vi "BehaviorControl.vi"() -> ()   [LabVIEW 2011]
uses:
  <instrlib>/niHWS/nihws.llb/niHWS Open File Permissions ID.ctl
  <vilib>/DAQmx/read.llb/DAQmx Read (Analog 1D Wfm NChan NSamp).vi
  <vilib>/DAQmx/create/channels.llb/DAQmx Create Channel (AI-Voltage-Basic).vi
  <vilib>/DAQmx/configure/timing.llb/DAQmx Timing (Sample Clock).vi
  <instrlib>/niHWS/nihws.llb/niHWS Write Analog DBL.vi
  <vilib>/DAQmx/miscellaneous.llb/DAQmx Fill In Error Info.vi
  <instrlib>/niHWS/nihws.llb/niHWS Write Analog WDT.vi
  <vilib>/vision/driver/NI_Vision_Acquisition_Software.lvlib
  <vilib>/ptbypt/NI_PtbyPt.lvlib
  C:/Program Files/National Instruments/LabVIEW 2011/resource/objmgr/imaqdx.rc
panel:
  in  "% Quality":i32=40
  out "Boolean":bool
  out "Command Sent":bool
  in  "Command":string
  in  "Port":u16=3000
  in  "Ephys":bool=TRUE
  in  "Video":bool=TRUE
  out "Ephys Recoding Signals":waveform(dbl)[](graph)
  in  "Camera":string(combo)
  in  "Video Modes":string(combo)="320x240 YUY2 30.00fps"
  in  "Compressor":string(combo)
  in  "Selected Path for AVI":path
  in  "Rec":bool
  out "fps":dbl format="%#_2g"
  in  "Start":bool
  out "Rec Time":dbl format="%#_3g"
  in  "stop":bool
  out "Image Out":T1(plugin-control)
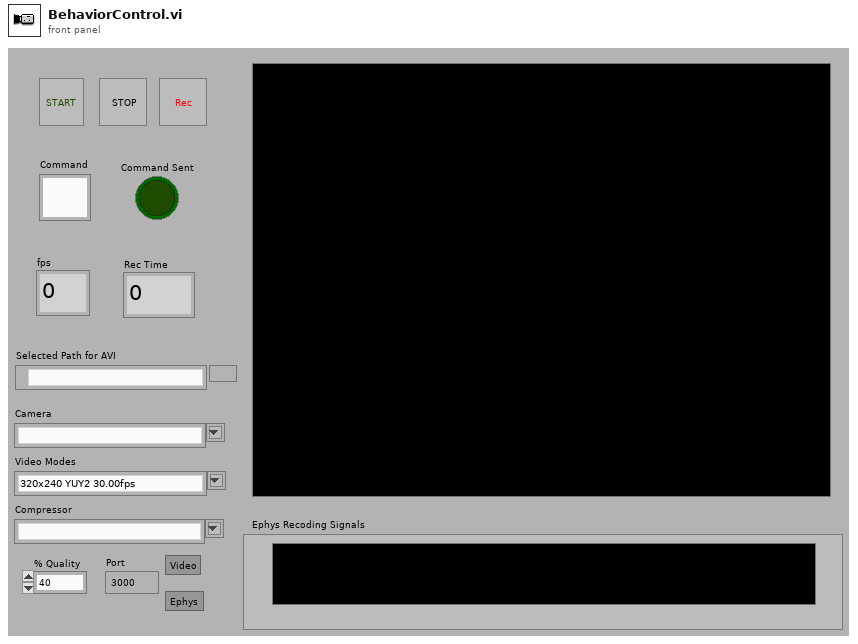
[diagram p1: front panel]
types:
  T1 = typedef "IMAQ Image.ctl" = refnum<image>
  T2 = typedef "niHWS Open File Permissions ID.ctl" = enum32{"Read Only", "Read/Write Existing", "Read/Write/Create New", "Read/Write/Create New Always"}
  T3 = cluster{"Type":u32, "Version":u32, "Flags":u32, "SerialNumberHigh":u32, "SerialNumberLow":u32, "BusType":u32, "InterfaceName":string, "VendorName":string, "ModelName":string, "CameraFileName":string, "CameraAttributeURL":string}[]
  T4 = cluster{"Type":u32, "Version":u32, "Flags":u32, "SerialNumberHigh":u32, "SerialNumberLow":u32, "BusType":u32, "InterfaceName":string, "VendorName":string, "ModelName":string, "CameraFileName":string, "CameraAttributeURL":string}
  T5 = typedef "IMAQdx.ctl" = refnum<k21>
  T6 = cluster{"Video Mode":u32, "Video Mode Name":string}[]
  T7 = typedef "AviRefnum.ctl" = refnum<k1>
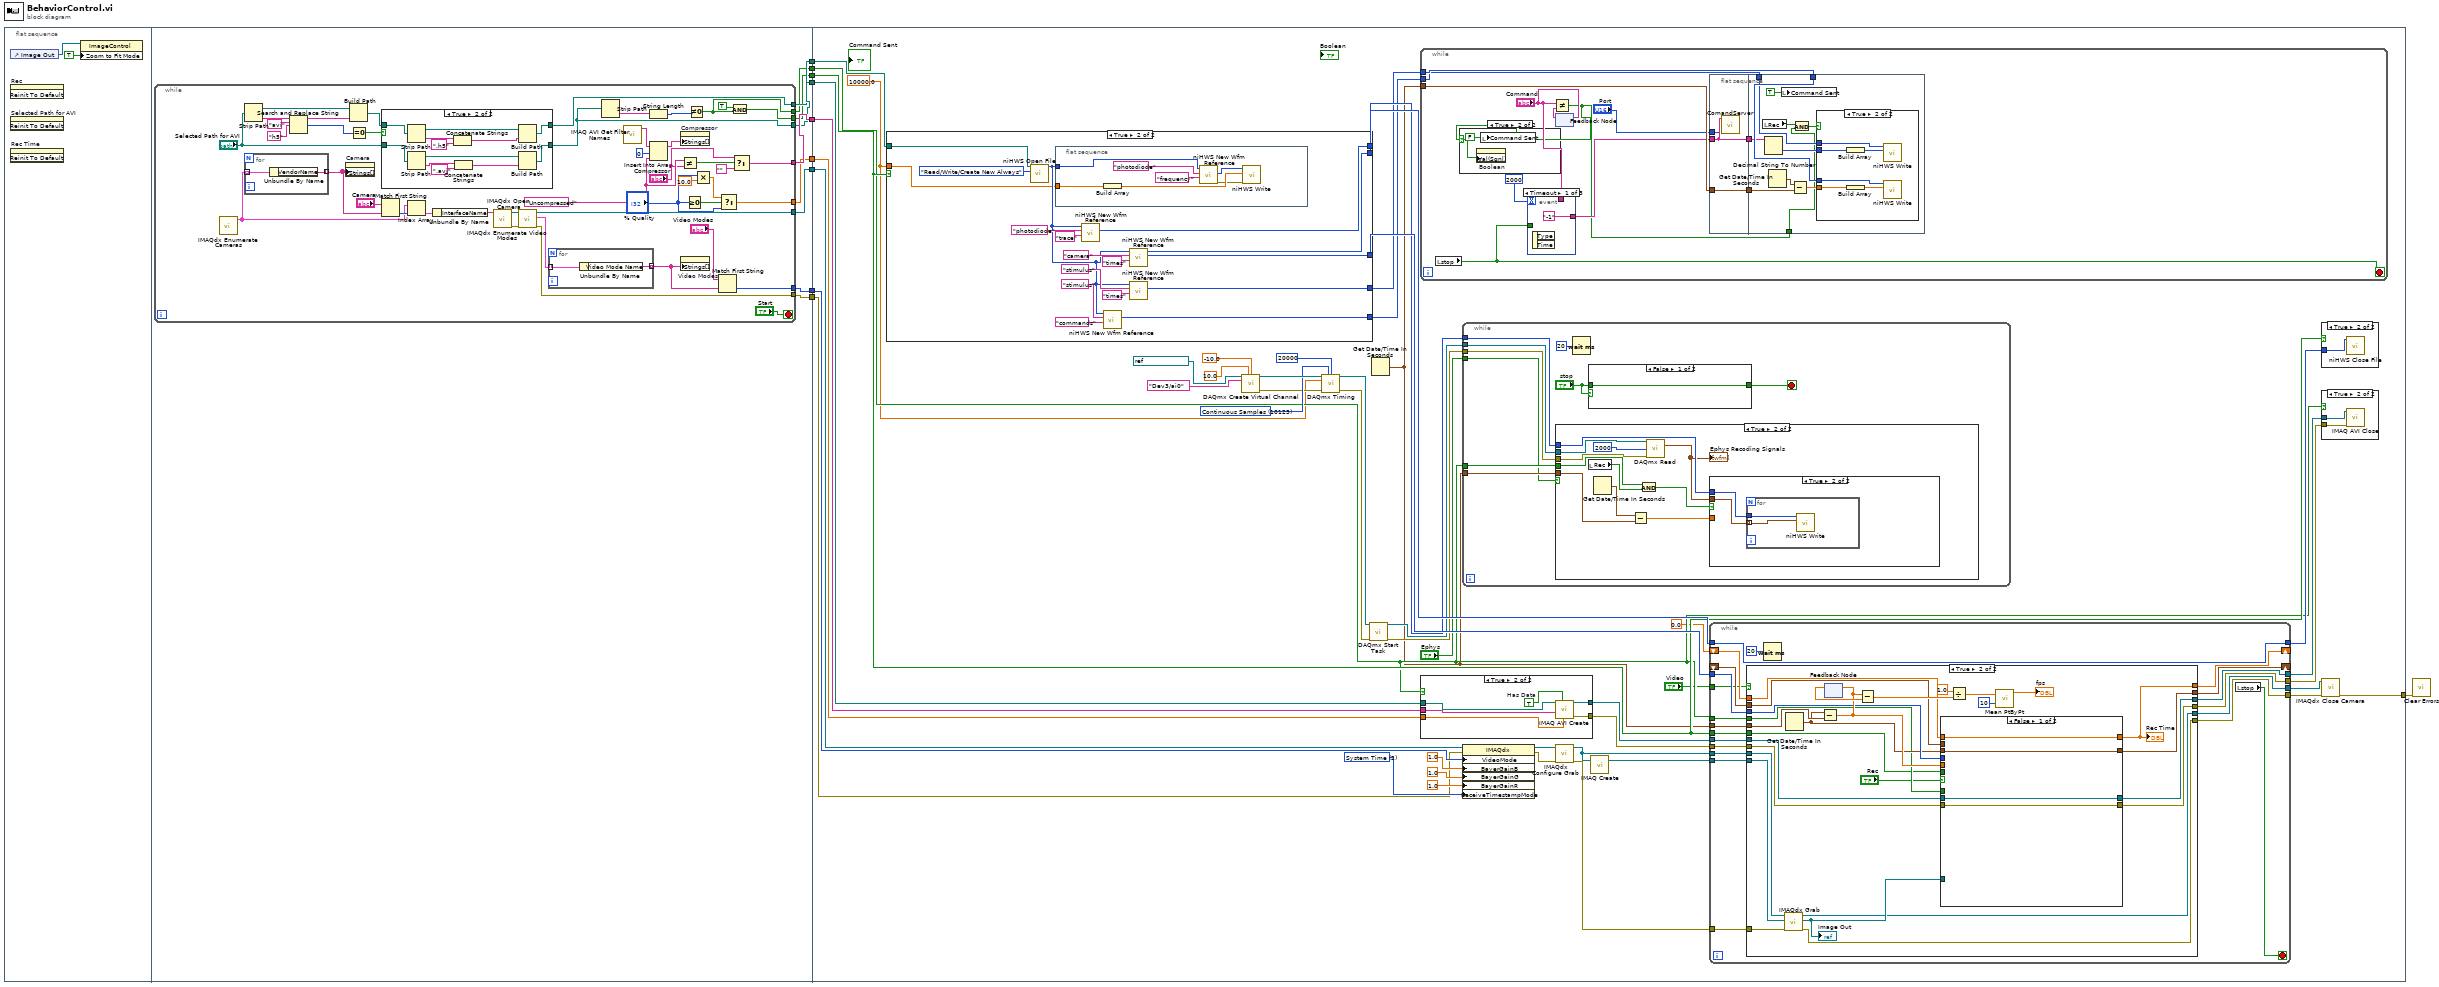
[diagram p0: block diagram]
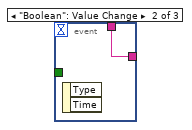
[diagram p4: hidden frame]
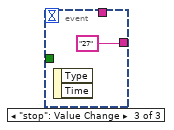
[diagram p5: hidden frame]
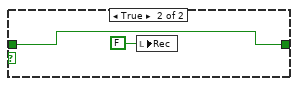
[diagram p9: hidden frame]
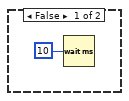
[diagram p14: hidden frame]
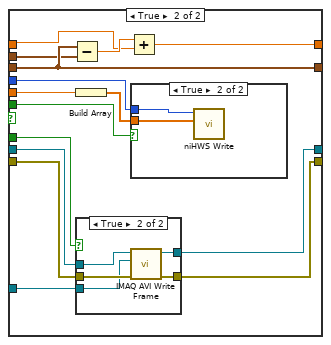
[diagram p15: hidden frame]
diagram:
  n1 = flat-sequence {
    tunnel: [w21] -> w10
    tunnel: [w20] -> w9
    tunnel: [w19] -> w8
    tunnel: [w18] -> w7
    tunnel: [w17] -> w6
    tunnel: [w16] -> w5
    tunnel: [w15] -> w4
    tunnel: [w14] -> w3
    tunnel: [w13] -> w2
    tunnel: w10 -> [w120]
    tunnel: w9 -> [w116]
    tunnel: w8 -> [w119]
    tunnel: w7 -> [w118]
    tunnel: w6 -> [w109]
    tunnel: w5 -> [w114]
    tunnel: w4 -> [w110]
    tunnel: w3 -> [w108]
    tunnel: w2 -> [w96]
    tunnel: [w90] -> w1
    frame #0 {
      n2 = control-ref of="Image Out"() -> (w12:refnum<vi>)
      n3 = invoke on="Rec" class="Bool (strict)" method="Reinit To Default"() -> ()  [unwired: 3 in, 3 out]
      n4 = invoke on="Selected Path for AVI" class="Path" method="Reinit To Default"() -> ()  [unwired: 3 in, 3 out]
      n5 = invoke on="Rec Time" class="DigNum (strict)" method="Reinit To Default"() -> ()  [unwired: 3 in, 3 out]
      n6 = property on="Property Node" class="ImageControl"(reference=w12, "Zoom to Fit Mode"=TRUE) -> ()  [unwired: 1 in, 2 out]
    }
    frame #1 {
      n7 = while {
        tunnel: [w46] -> w21
        tunnel: [w60] -> w20
        tunnel: [w37] -> w19
        tunnel: [w53] -> w18
        tunnel: [w27] -> w17
        tunnel: [w30] -> w16
        tunnel: [w45] -> w15
        tunnel: [w25] -> w14
        tunnel: [w26] -> w13
        stop <- "Start" stop-if-true
        w58 = "Uncompressed"
        n8 = call <vilib>:"IMAQdx Enumerate Cameras.vi"() -> ("Camera Information Array"=w49:T3)  [unwired: 10 in, 1 out]
        n9 = Strip Path(path="Selected Path for AVI") -> (stripped path=w44:path, name=w42:string)
        n10 = for {
          tunnel: w49 -> [w81] mode=indexing
          tunnel: [w80] -> w52 mode=indexing
          n11 = Unbundle By Name(w81) -> ("VendorName"=w80:string)
        }
        n12 = Search and Replace String(input string=w42, search string="avi", replace string="h5" ("replace string (\"\")")) -> (result string=w43:string, number of replacements=w33:i32)  [unwired: 5 in, 2 out]
        n13 = property on="Camera" class="CmbBox"("Strings[]"=w52) -> ()  [unwired: 2 in, 2 out]
        n14 = Build Path(base path=w44, name or relative path=w43) -> (appended path=w31:path)
        n15 = Equal To 0?(x=w33) -> (x = 0?=w32:bool)
        n16 = case shown="True" w32 {
          tunnel: "Selected Path for AVI" -> [w66 w79]
          tunnel: [w66 w78] -> w27
          tunnel: w31 -> [w67 w69]
          tunnel: [w67 w68] -> w30
          frame False {
          }
          frame True {
            n17 = Strip Path(path=w69) -> (stripped path=w73:path, name=w71:string)
            n18 = Strip Path(path=w79) -> (stripped path=w77:path, name=w75:string)
            n19 = Concatenate Strings(w71, ".h5" ("search string")) -> (w70:string)
            n20 = Concatenate Strings(w75, ".avi" ("search string")) -> (w74:string)
            n21 = Build Path(base path=w73, name or relative path=w70) -> (appended path=w68:path)
            n22 = Build Path(base path=w77, name or relative path=w74) -> (appended path=w78:path)
          }
        }
        n23 = Match First String(2:w52, 3:"Camera") -> (0:w50:i32)  [unwired: 1 out]
        n24 = Index Array(array=w49, index=w50) -> (element=w48:T4)
        n25 = Unbundle By Name(w48) -> ("InterfaceName"=w47:string)
        n26 = call <vilib>:"IMAQdx Open Camera.vi"("Session In"=w47) -> ("error out"=w64:errorcluster, "Session Out"=w65:T5)  [unwired: 9 in]
        n27 = call <vilib>:"IMAQdx Enumerate Video Modes.vi"("error in"=w64, "Session In"=w65) -> ("error out"=w45:errorcluster, "Video Modes"=w61:T6, "Session Out"=w46:T5)  [unwired: 6 in, 1 out]
        n28 = for {
          tunnel: w61 -> [w83] mode=indexing
          tunnel: [w82] -> w54 mode=indexing
          n29 = Unbundle By Name(w83) -> ("Video Mode Name"=w82:string)
        }
        n30 = Strip Path(path=w27) -> (name=w28:string)  [unwired: 1 out]
        n31 = call "IMAQ AVI Get Filter Names"() -> ("Filter Names"=w35:string[])  [unwired: 10 in, 1 out]
        n32 = String Length(string=w28) -> (length=w29:i32)
        n33 = Insert Into Array(array=w35, index=0 ("Index"), new element=w58) -> (w62:string[])
        n34 = property on="Compressor" class="CmbBox"("Strings[]"=w62) -> ()  [unwired: 2 in, 2 out]
        n35 = Not Equal?(x=w58, y="Compressor") -> (x != y?=w56:bool)
        n36 = property on="Video Modes" class="CmbBox"("Strings[]"=w54) -> ()  [unwired: 2 in, 2 out]
        n37 = Greater Or Equal To 0?(x="% Quality") -> (x >= 0?=w38:bool)
        n38 = Not Equal To 0?(x=w29) -> (x != 0?=w26:bool)
        n39 = Multiply(x="% Quality", y=10.0) -> (x*y=w39:dbl)
        n40 = Match First String(2:w54, 3:"Video Modes") -> (0:w53:i32)  [unwired: 1 out]
        n41 = Select(t=w39, s=w38, f="% Quality") -> (s? t:f=w37:dbl)
        n42 = And(x=TRUE, y=w26) -> (x .and. y?=w25:bool)
        n43 = Select(t="Compressor", s=w56, f="") -> (s? t:f=w60:string)
      }
    }
    frame #2 {
      w103 = 10123 items=["Finite Samples"=10178, "Continuous Samples"=10123, "Hardware Timed Single Point"=12522] ("sample mode")
      w84 = 10000.0 ("rate")
      w115 = u32 2 items=["None", "Tick Count", "System Time"] ("ReceiveTimestampMode")
      n44 = case shown="True" w108 {
        tunnel: w114 -> [_ w218]
        tunnel: [_ w217] -> w113
        tunnel: [_ w216] -> w112
        tunnel: [_ w215] -> w107
        tunnel: [_ w208] -> w86
        tunnel: [_ w207] -> w85
        tunnel: w84 -> [_ w205]
        frame False {
        }
        frame True {
          n45 = call <instrlib>:"niHWS Open File.vi"("permissions (0:read only)"=niHWS_Open_File_Permissions_ID."Read/Write/Create New Always", "file path"=w218) -> ("file handle"=w206:u32)  [unwired: 8 in, 1 out]
          n46 = flat-sequence {
            tunnel: w205 -> [w224]
            tunnel: w206 -> [w223]
            frame #0 {
              n47 = Build Array(w224) -> (w225:dbl[])
              n48 = call <instrlib>:"niHWS New Wfm Reference.vi"("waveform name (empty)"="frequency" ("group name (empty)"), "group name (empty)"="photodiode", "file handle in"=w223) -> ("error out"=w222:errorcluster, "waveform reference"=w228:u32)  [unwired: 6 in, 1 out]
              n49 = call-poly <instrlib>:"niHWS Write.vi"("error in (no error)"=w222, "data"=w225, "waveform reference in"=w228) -> ()  [unwired: 7 in, 2 out]
            }
          }
          n50 = call <instrlib>:"niHWS New Wfm Reference.vi"("waveform name (empty)"="trace", "group name (empty)"="photodiode", "file handle in"=w206) -> ("waveform reference"=w215:u32)  [unwired: 6 in, 2 out]
          n51 = call <instrlib>:"niHWS New Wfm Reference.vi"("waveform name (empty)"="commands" ("group name (empty)"), "group name (empty)"="stimulus", "file handle in"=w206) -> ("waveform reference"=w207:u32)  [unwired: 6 in, 2 out]
          n52 = call <instrlib>:"niHWS New Wfm Reference.vi"("waveform name (empty)"="times" ("group name (empty)"), "group name (empty)"="camera", "file handle in"=w206) -> ("waveform reference"=w217:u32, "file handle out"=w216:u32)  [unwired: 6 in, 1 out]
          n53 = call <instrlib>:"niHWS New Wfm Reference.vi"("waveform name (empty)"="times" ("group name (empty)"), "group name (empty)"="stimulus", "file handle in"=w206) -> ("waveform reference"=w208:u32)  [unwired: 6 in, 2 out]
        }
      }
      n54 = call-poly <vilib>:"DAQmx Create Virtual Channel.vi"("task in"=refnum<k21> "PHOTODIODE", "maximum value"=10.0, "minimum value"=-10.0, "physical channels"=tag "Dev3/ai0") -> ("task out"=w104:refnum<k21>, "error out"=w101:errorcluster)  [unwired: 10 in]
      n55 = call-poly <vilib>:"DAQmx Timing.vi"("task/channels in"=w104, "sample mode"=w103, "samples per channel"=20000, "rate"=w84, "error in"=w101) -> ("task out"=w98:refnum<k21>, "error out"=w97:errorcluster)  [unwired: 9 in]
      n56 = call <vilib>:"DAQmx Start Task.vi"("task/channels in"=w98, "error in"=w97) -> ("task out"=w100:refnum<k21>, "error out"=w99:errorcluster)  [unwired: 12 in]
      n57 = Get Date/Time In Seconds() -> (seconds since 1Jan1904=w87:timestamp)
      n58 = while {
        tunnel: w87 -> [w143]
        tunnel: w86 -> [w142]
        tunnel: w85 -> [w141]
        stop <- w132 stop-if-true
        n59 = local read "stop"() -> (w132:bool)
        n60 = event shown="[0] Timeout" {
          selector: _ -> [_ _ _]
          dyn-events: _ -> [_ _ _]
          timeout: 2000 -> [_ _ _]
          tunnel: ["-1" ("f") w147 "27"] -> w135
          tunnel: "Command" -> [_ w147 _]
          tunnel: w132 -> [_ _ _]
          event Timeout {
            n61 = event-data() -> ()  [unwired: 1 in, 2 out]
          }
          event "Boolean": Value Change {
            n62 = event-data() -> ()  [unwired: 1 in, 2 out]
          }
          event "stop": Value Change {
            n63 = event-data() -> ()  [unwired: 1 in, 2 out]
          }
        }
        n64 = feedback-in #1("Command") -> ()
        n65 = feedback #1() -> (w139:string)  [unwired: 1 in]
        n66 = Not Equal?(x="Command", y=w139) -> (x != y?=w133:bool)
        n67 = case shown="True" w133 {
          selector: w133 -> [_ w145]
          frame False {
          }
          frame True {
            n68 = property on="Boolean" class="Bool (strict)"("Val(Sgnl)"=w145) -> ()  [unwired: 2 in, 2 out]
            n69 = local write "Command Sent"(FALSE ("Command Completed")) -> ()
          }
        }
        n70 = flat-sequence {
          tunnel: [w151] -> w138
          tunnel: [w150] -> w137
          tunnel: "Port" -> [w149]
          tunnel: w143 -> [w151]
          tunnel: w135 -> [w150]
          tunnel: w138 -> [w161]
          tunnel: w142 -> [w160]
          tunnel: w137 -> [w155]
          tunnel: w141 -> [w158]
          tunnel: w133 -> [w152]
          frame #0 {
            n71 = call "ComandServer.vi"("Port"=w149, "Input"=w150) -> ()  [unwired: 8 in, 2 out]
          }
          frame #1 {
            n72 = local read "Rec"() -> (w154:bool)
            n73 = Decimal String To Number(string=w155) -> (number=w156:i32)  [unwired: 2 in, 1 out]
            n74 = Get Date/Time In Seconds() -> (seconds since 1Jan1904=w162:timestamp)
            n75 = local write "Command Sent"(TRUE ("Command Completed")) -> ()
            n76 = Subtract(x=w162, y=w161) -> (x-y=w159:dbl)
            n77 = And(x=w154, y=w152) -> (x .and. y?=w153:bool)
            n78 = case shown="True" w153 {
              tunnel: w160 -> [_ w168]
              tunnel: w159 -> [_ w167]
              tunnel: w156 -> [_ w164]
              tunnel: w158 -> [_ w163]
              frame False {
              }
              frame True {
                n79 = Build Array(w164) -> (w165:i32[])
                n80 = Build Array(w167) -> (w166:dbl[])
                n81 = call-poly <instrlib>:"niHWS Write.vi"("data"=w165, "waveform reference in"=w163) -> ()  [unwired: 8 in, 2 out]
                n82 = call-poly <instrlib>:"niHWS Write.vi"("data"=w166, "waveform reference in"=w168) -> ()  [unwired: 8 in, 2 out]
              }
            }
          }
        }
      }
      n83 = case shown="True" w96 {
        tunnel: [_ w202] -> w131
        tunnel: [_ w201] -> w128
        tunnel: w119 -> [_ w200]
        tunnel: w116 -> [_ w199]
        tunnel: w109 -> [_ w198]
        frame False {
        }
        frame True {
          w203 = TRUE  # Has Data
          n84 = call "IMAQ AVI Create"("quality"=w200, "Has Data"=w203, "Compression Filter"=w199, "AVI Path"=w198) -> ("error out"=w201:errorcluster, "Avi Refnum"=w202:T7)  [unwired: 3 in, 3 out]
        }
      }
      n85 = while {
        tunnel: w107 -> [w177]
        tunnel: w100 -> [w176]
        tunnel: w99 -> [w175]
        tunnel: w87 -> [w174]
        tunnel: w96 -> [w172]
        tunnel: "Ephys" -> [w169]
        stop <- w170 stop-if-true
        n86 = case shown="True" w169 {
          tunnel: w177 -> [_ w188]
          tunnel: w176 -> [_ w186]
          tunnel: w175 -> [_ w185]
          tunnel: w174 -> [_ w182]
          tunnel: w172 -> [_ w180]
          frame False {
          }
          frame True {
            n87 = local read "Rec"() -> (w179:bool)
            n88 = Get Date/Time In Seconds() -> (seconds since 1Jan1904=w183:timestamp)
            n89 = Subtract(x=w183, y=w182) -> (x-y=w181:dbl)
            n90 = And(x=w180, y=w179) -> (x .and. y?=w178:bool)
            n91 = call-poly <vilib>:"DAQmx Read.vi"("task/channels in"=w186, "number of samples per channel"=2000, "error in"=w185) -> ("data"=w184:waveform(dbl)[])  [unwired: 10 in, 2 out]
            "Ephys Recoding Signals" <- w184
            n92 = case shown="True" w178 {
              tunnel: w188 -> [_ w190]
              tunnel: w184 -> [_ w189]
              tunnel: w181 -> [_ _]
              frame False {
              }
              frame True {
                n93 = for {
                  tunnel: w190 -> [w192]
                  tunnel: w189 -> [w191] mode=indexing
                  n94 = call-poly <instrlib>:"niHWS Write.vi"("analog waveform"=w191, "waveform reference in"=w192) -> ()  [unwired: 8 in, 2 out]
                }
              }
            }
          }
        }
        n95 = Wait (ms)(milliseconds to wait=u32 20) -> ()  [unwired: 1 out]
        n96 = case shown="False" "stop" {
          tunnel: "stop" -> [w193 w194]
          tunnel: [w193 w194] -> w170
          frame False {
          }
          frame True {
            n97 = local write "Rec"(FALSE ("Rec")) -> ()
          }
        }
      }
      n98 = property class="IMAQdx"(reference=w120, error in=w110, "VideoMode"=w118, "BayerGainB"=1.0, "BayerGainG"=1.0, "BayerGainR"=1.0, "ReceiveTimestampMode"=w115) -> (reference out=w122:T5, error out=w121:errorcluster)
      n99 = call <vilib>:"IMAQdx Configure Grab.vi"("error in"=w121, "Session In"=w122) -> ("error out"=w126:errorcluster, "Session Out"=w117:T5)  [unwired: 8 in]
      n100 = call "IMAQ Create"("Image Name"=w117) -> ("New Image"=w127:T1)  [unwired: 4 in, 1 out]
      n101 = while {
        tunnel: [w249] -> w130
        tunnel: [w248] -> w129
        tunnel: w131 -> [w247]
        tunnel: w128 -> [w246]
        tunnel: w127 -> [w237]
        tunnel: w117 -> [w238]
        tunnel: w126 -> [w236]
        tunnel: w87 -> [w245]
        tunnel: w113 -> [w244]
        tunnel: w112 -> [w243]
        tunnel: [w243] -> w111
        shift-right: [w242] -> _
        shift-left: _ -> [w241]
        tunnel: w108 -> [w239]
        tunnel: w96 -> [w240]
        tunnel: [w235] -> w95
        tunnel: [w234] -> w94
        shift-right: [w232] -> _
        shift-left: 0.0 -> [w233]
        tunnel: "Video" -> [w231]
        stop <- w230 stop-if-true
        n102 = case shown="True" w231 {
          tunnel: [_ w277] -> w249
          tunnel: [_ w276] -> w248
          tunnel: w247 -> [_ w275]
          tunnel: w246 -> [_ w274]
          tunnel: w245 -> [_ w273]
          tunnel: w244 -> [_ w267]
          tunnel: [_ w265] -> w242
          tunnel: w241 -> [_ w264]
          tunnel: w240 -> [_ w262]
          tunnel: w239 -> [_ w261]
          tunnel: w238 -> [_ w259]
          tunnel: w237 -> [_ w258]
          tunnel: w236 -> [_ w257]
          tunnel: [_ w256] -> w235
          tunnel: [_ w255] -> w234
          tunnel: w233 -> [_ w254]
          tunnel: [_ w253] -> w232
          frame False {
            n103 = Wait (ms)(milliseconds to wait=u32 10) -> ()  [unwired: 1 out]
          }
          frame True {
            n104 = call <vilib>:"IMAQdx Grab.vi"("error in"=w257, "Image In"=w258, "Session In"=w259) -> ("error out"=w255:errorcluster, "Image Out"=w260:T1, "Session Out"=w256:T5)  [unwired: 5 in, 1 out]
            "Image Out" <- w260
            n105 = Get Date/Time In Seconds() -> (seconds since 1Jan1904=w266:timestamp)
            n106 = Subtract(x=w266, y=w273) -> (x-y=w268:dbl)
            n107 = feedback #2() -> (w272:dbl)  [unwired: 1 in]
            n108 = feedback-in #2(w268) -> ()
            n109 = Subtract(x=w268, y=w272) -> (x-y=w270:dbl)
            n110 = case shown="False" "Rec" {
              tunnel: [w280 w296] -> w277
              tunnel: [w281 w295] -> w276
              tunnel: w275 -> [w280 w294]
              tunnel: w274 -> [w281 w293]
              tunnel: w260 -> [_ w292]
              tunnel: [w278 w282] -> w253
              tunnel: w268 -> [_ w291]
              tunnel: w267 -> [_ w289]
              tunnel: [w279 w287] -> w265
              tunnel: w266 -> [w279 w287]
              tunnel: w264 -> [_ w286]
              tunnel: w261 -> [_ w285]
              tunnel: w262 -> [_ w284]
              tunnel: w254 -> [w278 w283]
              frame False {
              }
              frame True {
                n111 = Subtract(x=w287, y=w286) -> (x-y=w288:dbl)
                n112 = Build Array(w291) -> (w290:dbl[])
                n113 = case shown="True" w284 {
                  tunnel: [_ w301] -> w296
                  tunnel: [_ w300] -> w295
                  tunnel: w294 -> [_ w299]
                  tunnel: w293 -> [_ w298]
                  tunnel: w292 -> [_ w297]
                  frame False {
                  }
                  frame True {
                    n114 = call "IMAQ AVI Write Frame"("error in (no error)"=w298, "Image"=w297, "Avi Refnum"=w299) -> ("error out"=w300:errorcluster, "Avi Refnum (duplicate)"=w301:T7)  [unwired: 7 in]
                  }
                }
                n115 = Add(x=w288, y=w283) -> (x+y=w282:dbl)
                n116 = case shown="True" w285 {
                  tunnel: w290 -> [_ w303]
                  tunnel: w289 -> [_ w302]
                  frame False {
                  }
                  frame True {
                    n117 = call-poly <instrlib>:"niHWS Write.vi"("data"=w303, "waveform reference in"=w302) -> ()  [unwired: 8 in, 2 out]
                  }
                }
              }
            }
            "Rec Time" <- w253
            n118 = Divide(x=1.0, y=w270) -> (x/y=w269:dbl)
            n119 = call <vilib>:"Mean PtByPt.vi"("x"=w269, "sample length"=10) -> ("mean"=→"fps":dbl)  [unwired: 2 in, 1 out]
          }
        }
        n120 = Wait (ms)(milliseconds to wait=u32 20) -> ()  [unwired: 1 out]
        n121 = local read "stop"() -> (w230:bool)
      }
      n122 = case shown="True" w108 {
        tunnel: w111 -> [_ w204]
        frame False {
        }
        frame True {
          n123 = call <instrlib>:"niHWS Close File.vi"("file handle"=w204) -> ()  [unwired: 10 in, 1 out]
        }
      }
      n124 = case shown="True" w96 {
        tunnel: w130 -> [_ w197]
        tunnel: w129 -> [_ w196]
        frame False {
        }
        frame True {
          n125 = call "IMAQ AVI Close"("error in (no error)"=w196, "Avi Refnum"=w197) -> ()  [unwired: 9 in, 1 out]
        }
      }
      n126 = call <vilib>:"IMAQdx Close Camera.vi"("error in"=w94, "Session In"=w95) -> ("error out"=w90:errorcluster)  [unwired: 9 in]
    }
  }
  n127 = call <vilib>:"Clear Errors.vi"("error in (no error)"=w1) -> ()  [unwired: 6 in, 1 out]
